vi "rsspecan read trace example_test2.vi"() -> ()   [LabVIEW 2011]
doc: "This VI shows how to query the trace from Rohde&Schwarz analyzer, supported by latest rsspecan attribute-based instrument driver. Before running the example, specify VISA resource name and properly set ID Query and Reset Device booleans. After running the example, select proper center frequency and frequency span and pres Start button to show the trace in graph."
uses:
  <vilib>/Utility/file.llb/Write To Spreadsheet File (DBL).vi
panel:
  out "XY Graph":cluster{dbl[], "Amplitude":dbl[]}(graph)
  out "Points":i32=5001
  in  "file path (dialog if empty)":path=path "C:/Users/VGroup/Desktop/PNA data/20140521/EOM beat"
  in  "Trace (1)":i32=1
  in  "Stop":bool
  out "Frequency Spectrum":dbl[](graph)
  in  "Start":bool
  in  "Center Frequency":dbl=10000000.0 format="%^.3e"
  in  "Span":dbl=20000000.0 format="%^.3e"
  in  "Exit":bool
  in  "ID Query":bool=TRUE
  in  "Reset Device":bool
  in  "VISA resource name":refnum<visa-resource-name>="GPIB::20"
  # "Rohde & Schwarz Spectrum Analyzer\nRead Trace Example"
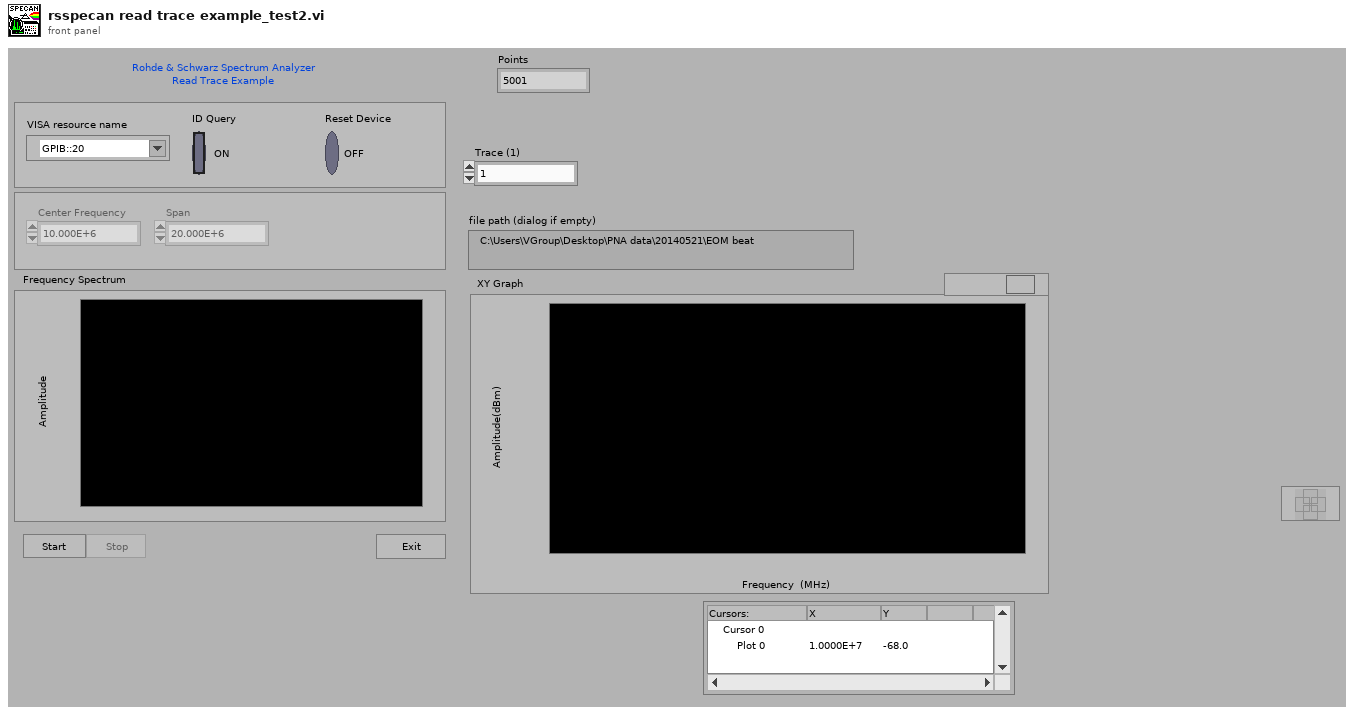
[diagram p1: front panel]
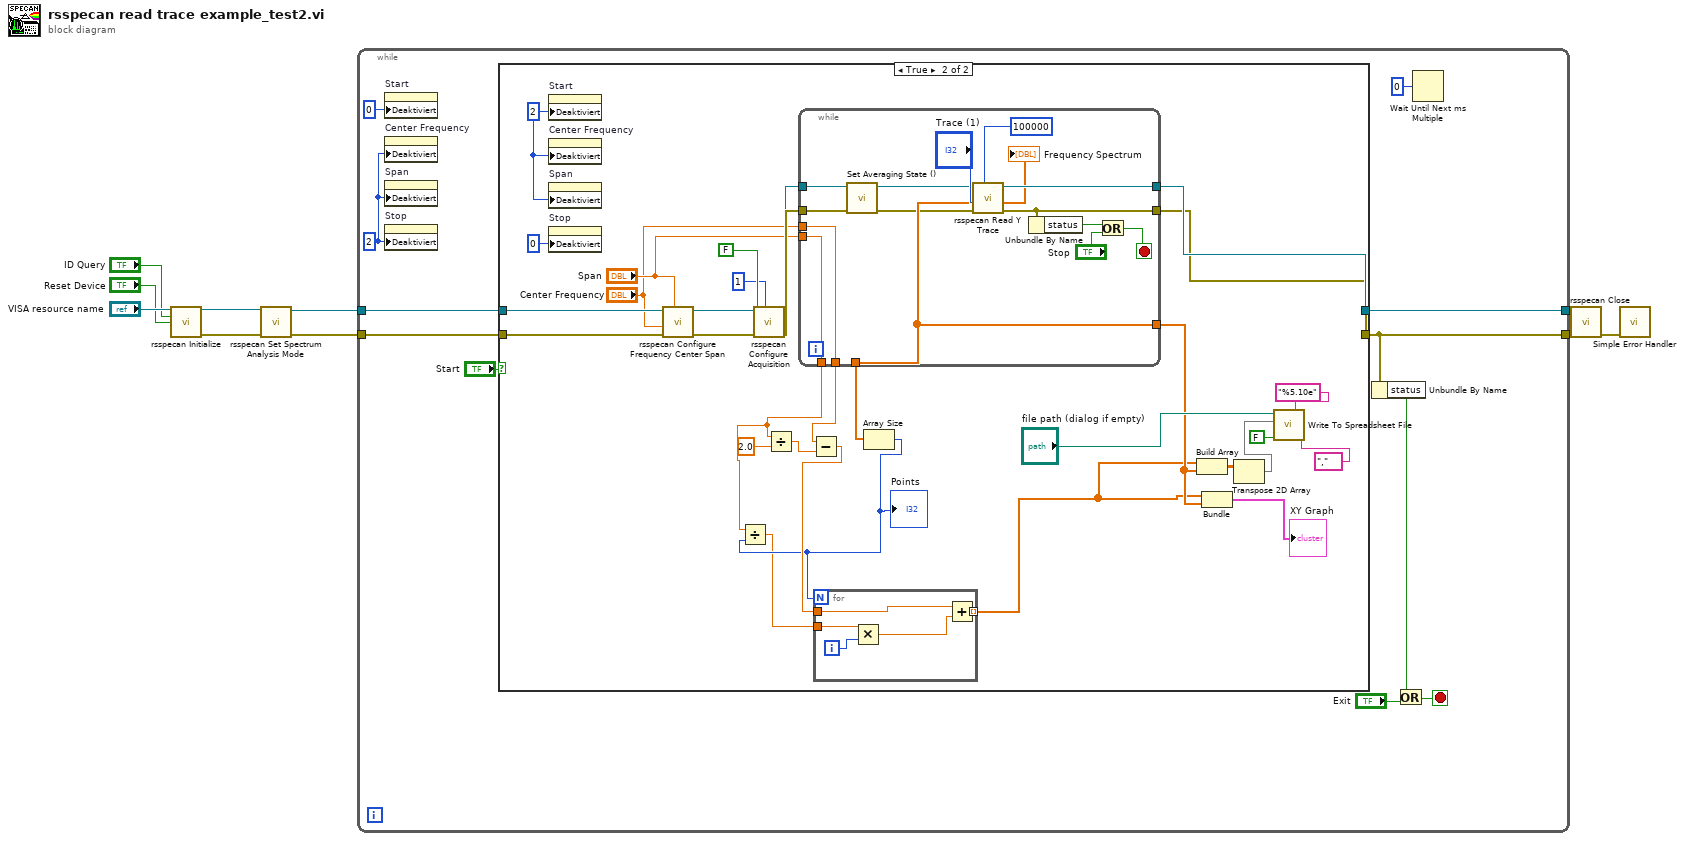
[diagram p0: block diagram]
diagram:
  n1 = call <instrlib>:"rsspecan Initialize.vi"("VISA resource name"="VISA resource name", "ID Query (T: Check)"="ID Query", "Reset (T: Reset)"="Reset Device") -> ("VISA resource name out"=w5:refnum<visa-resource-name>, "error out"=w4:errorcluster)  [unwired: 1 in, 10 out]
  n2 = call <instrlib>:"rsspecan Set Spectrum Analysis Mode.vi"("error in (no error)"=w4, "VISA resource name"=w5) -> ("error out"=w2:errorcluster, "VISA resource name out"=w1:refnum<visa-resource-name>)  [unwired: 8 out]
  n3 = while {
    tunnel: w1 -> [w21]
    tunnel: w2 -> [w20]
    tunnel: [w17] -> w7
    tunnel: [w16] -> w6
    stop <- w15 stop-if-true
    w11 = u8 2 ("Disabled")
    n4 = property on="Start" class="Bool"("Deaktiviert"=u8 0 ("Disabled")) -> ()  [unwired: 2 in, 2 out]
    n5 = property on="Center Frequency" class="DigNum (strict)"("Deaktiviert"=w11) -> ()  [unwired: 2 in, 2 out]
    n6 = property on="Span" class="DigNum (strict)"("Deaktiviert"=w11) -> ()  [unwired: 2 in, 2 out]
    n7 = property on="Stop" class="Bool"("Deaktiviert"=w11) -> ()  [unwired: 2 in, 2 out]
    n8 = case shown="True" "Start" {
      tunnel: w21 -> [w23 w54]
      tunnel: w20 -> [w22 w53]
      tunnel: [w23 w50] -> w17
      tunnel: [w22 w49] -> w16
      frame False {
      }
      frame True {
        w52 = u8 2 ("Disabled")
        n9 = property on="Start" class="Bool"("Deaktiviert"=w52) -> ()  [unwired: 2 in, 2 out]
        n10 = property on="Center Frequency" class="DigNum (strict)"("Deaktiviert"=w52) -> ()  [unwired: 2 in, 2 out]
        n11 = property on="Span" class="DigNum (strict)"("Deaktiviert"=w52) -> ()  [unwired: 2 in, 2 out]
        n12 = property on="Stop" class="Bool"("Deaktiviert"=u8 0 ("Disabled")) -> ()  [unwired: 2 in, 2 out]
        n13 = call <instrlib>:"rsspecan Configure Frequency Center Span.vi"("Span"="Span", "error in (no error)"=w53, "Center Frequency"="Center Frequency", "VISA resource name"=w54) -> ("error out"=w48:errorcluster, "VISA resource name out"=w47:refnum<visa-resource-name>)  [unwired: 1 in, 5 out]
        n14 = call <instrlib>:"rsspecan Configure Acquisition.vi"("Number Of Sweeps (1)"=1 ("Number Of Sweeps (0)"), "error in (no error)"=w48, "Sweep Mode Continuous (Off)"=FALSE, "VISA resource name"=w47) -> ("error out"=w45:errorcluster, "VISA resource name out"=w44:refnum<visa-resource-name>)  [unwired: 1 in, 5 out]
        n15 = while {
          tunnel: w44 -> [w65]
          tunnel: w45 -> [w63]
          tunnel: [w72] -> w50
          tunnel: [w70] -> w49
          tunnel: [w66] -> w27
          tunnel: [w66] -> w37
          tunnel: "Span" -> [w61]
          tunnel: [w61] -> w32
          tunnel: "Center Frequency" -> [w60]
          tunnel: [w60] -> w35
          stop <- w71 stop-if-true
          n16 = call "Set Averaging State ()"("error in (no error)"=w63, "instrument handle"=w65) -> ("error out"=w62:errorcluster, "instrument handle out"=w64:refnum<visa-resource-name>)  [unwired: 8 in]
          n17 = call <instrlib>:"rsspecan Read Y Trace.vi"("Maximum Time (5000)"=u32 100000, "error in (no error)"=w62, "Trace (1)"="Trace (1)", "VISA resource name"=w64) -> ("error out"=w70:errorcluster, "Amplitude"=w66:dbl[], "VISA resource name out"=w72:refnum<visa-resource-name>)  [unwired: 1 in, 4 out]
          "Frequency Spectrum" <- w66
          n18 = Unbundle By Name(w70) -> ("status"=w69:bool)
          n19 = Or(x=w69, y="Stop") -> (x .or. y?=w71:bool)
        }
        n20 = Divide(x=w32, y=2.0) -> (x/y=w34:dbl)
        n21 = Subtract(x=w35, y=w34) -> (x-y=w33:dbl)
        n22 = Array Size(array=w37) -> (size(s)=w31:i32)
        "Points" <- w31
        n23 = Divide(x=w32, y=w31) -> (x/y=w30:dbl)
        n24 = for {
          N: w31 -> [_]
          tunnel: w33 -> [w59]
          tunnel: [w58] -> w24 mode=indexing
          tunnel: w30 -> [w56]
          i -> [w57]
          n25 = Multiply(x=w56, y=w57) -> (x*y=w55:dbl)
          n26 = Add(x=w59, y=w55) -> (x+y=w58:dbl)
        }
        n27 = Build Array(w24, w27) -> (w26:dbl[][])
        n28 = Bundle(w24, "Amplitude"=w27) -> (→"XY Graph":cluster{dbl[], "Amplitude":dbl[]})  [unwired: 1 in]
        n29 = Transpose 2D Array(2D array=w26) -> (transposed array=w25:dbl[][])
        n30 = call-poly <vilib>:"Write To Spreadsheet File.vi"("delimiter (\\t)"="," ("delimiter (Tab)"), "format (%.3f)"="%5.10e", "append to file? (new file:F)"=FALSE, "2D data"=w25, "file path (dialog if empty)"="file path (dialog if empty)") -> ()  [unwired: 3 in, 1 out]
      }
    }
    n31 = Unbundle By Name(w16) -> ("status"=w13:bool)
    n32 = Or(x=w13, y="Exit") -> (x .or. y?=w15:bool)
    n33 = Wait Until Next ms Multiple(millisecond multiple=u32 0) -> ()  [unwired: 1 out]
  }
  n34 = call <instrlib>:"rsspecan Close.vi"("error in (no error)"=w6, "VISA resource name"=w7) -> ("error out"=w3:errorcluster)  [unwired: 9 out]
  n35 = call <vilib>:"Simple Error Handler.vi"("error in (no error)"=w3) -> ()  [unwired: 1 in, 8 out]
